vi "resonant.piezo.config.vi"() -> (3 "appended array":dbl[][](array[numeric]))   [LabVIEW 2012]
uses:
  GFG/GFGnumericGet.vi
  GFG/GFGbooleanGet.vi
  GFG/GFG library.lvlib
panel:
  out "pockels cell control":dbl[](graph)
  out "piezo control":dbl[](graph)
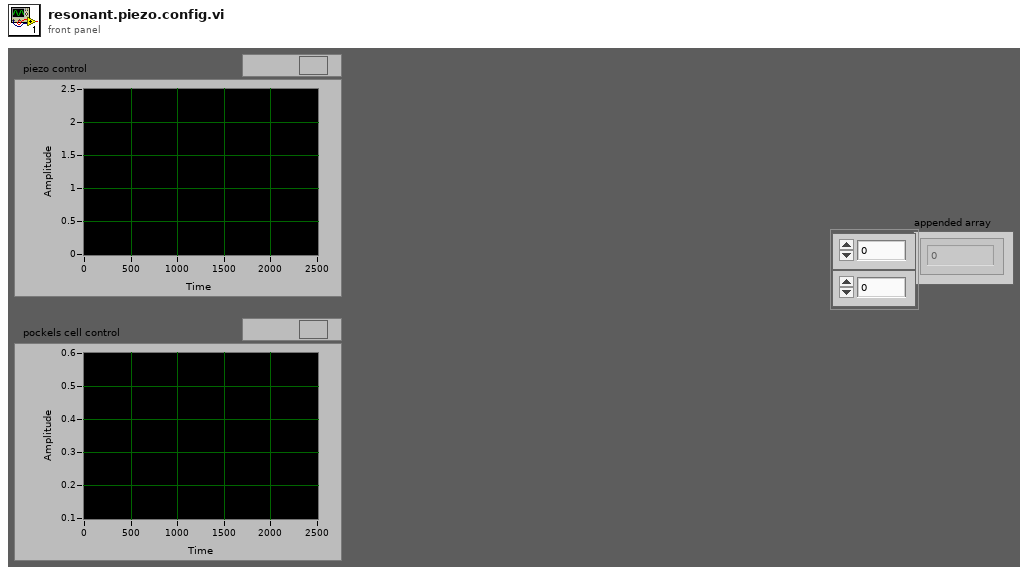
[diagram p1: front panel]
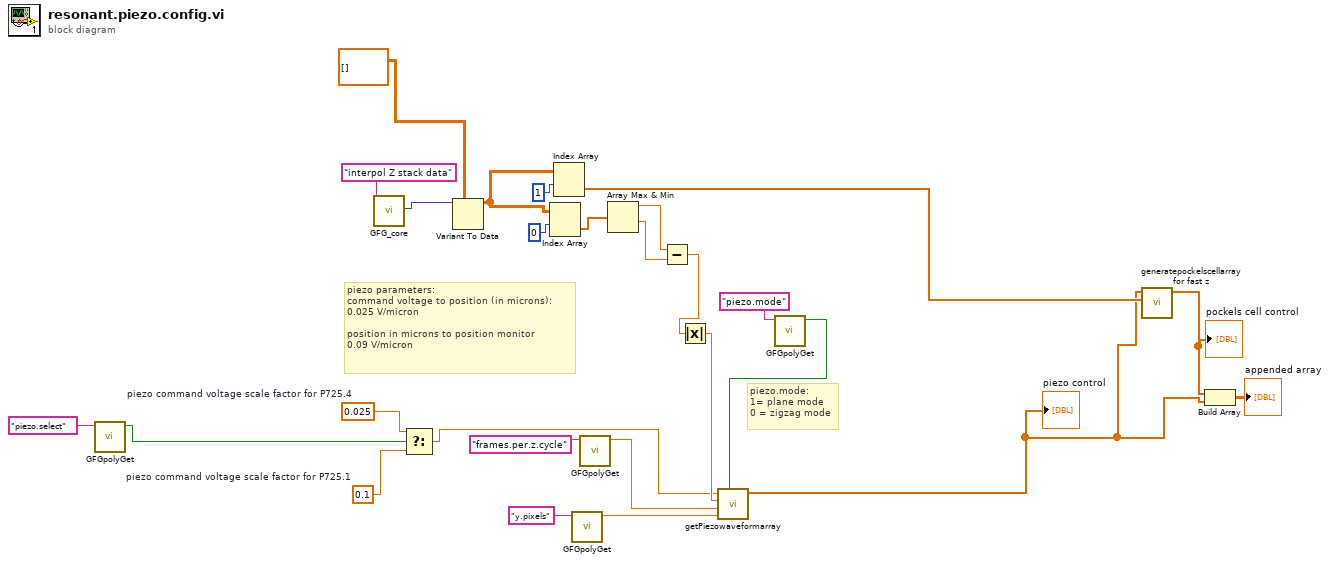
[diagram p0: block diagram]
diagram:
  w4 = 0.1  # piezo command voltage scale factor for P725.1
  w5 = 0.025  # piezo command voltage scale factor for P725.4
  # "piezo.mode: \n1= plane mode\n0 = zigzag mode"
  # "piezo parameters:\ncommand voltage to position (in microns):\n0.025 V/micron\n\nposition in microns to position monitor\n0.09 V/micron"
  n1 = call-poly "GFGpolyGet.vi"("Variable Name in"="piezo.select") -> ("Boolean"=w2:bool)  [unwired: 10 in]
  n2 = call "GFG_core.vi"("Variable Name in"="interpol Z stack data") -> ("Variant Out"=w22:variant)  [unwired: 12 in, 6 out]
  n3 = Select(t=w5, s=w2, f=w4) -> (s? t:f=w1:dbl)
  n4 = Variant To Data(type=dbl[][] [] ("Interpolated Data"), Variant=w22) -> (data=w19:dbl[][])  [unwired: 1 in, 1 out]
  n5 = Index Array(array=w19, index (row)=0 ("disabled index (col)")) -> (element=w18:dbl[])  [unwired: 1 in]
  n6 = Index Array(array=w19, index (row)=1 ("disabled index (col)")) -> (element=w20:dbl[])  [unwired: 1 in]
  n7 = call-poly "GFGpolyGet.vi"("Variable Name in"="y.pixels") -> ("Numeric"=w8:dbl)  [unwired: 9 in, 1 out]
  n8 = call-poly "GFGpolyGet.vi"("Variable Name in"="frames.per.z.cycle" ("Tag in")) -> ("Numeric"=w12:dbl)  [unwired: 9 in, 1 out]
  n9 = Array Max & Min(array=w18) -> (max value=w17:dbl, min value=w16:dbl)  [unwired: 2 out]
  n10 = Subtract(x=w17, y=w16) -> (x-y=w15:dbl)
  n11 = Absolute Value(x=w15) -> (abs(x)=w14:dbl)
  n12 = call-poly "GFGpolyGet.vi"("Variable Name in"="piezo.mode" ("Tag in")) -> ("Boolean"=w24:bool)  [unwired: 10 in]
  n13 = call "getPiezowaveformarray.vi"("planes or zigzag"=w24, "pixel.num"=w8, "frames.per.z.cycle"=w12, "total.z.distance"=w14, "piezo scale factor"=w1) -> ("Array"=w9:dbl[])  [unwired: 6 in]
  "piezo control" <- w9
  n14 = call "generatepockelscellarray for fast z.vi"("interpolated pockels cell data"=w20, "piezo control"=w9) -> ("pockelscellarray"=w23:dbl[])  [unwired: 9 in]
  "pockels cell control" <- w23
  n15 = Build Array(w23, w9) -> (→"appended array":dbl[][])
